vi "Configure Switcher Sweep Input.vi"(0 "VISA resource name":refnum<visa-resource-name>, 1 "Network Name (0)":string="0", 2 "Switch Number Of Steps (0)":i32, 5 "Channel (0: Channel A)":i32(ring) items=["Channel A", "Channel B"], 7 "Enable Input Switch (T: Enable)":bool=TRUE, 9 "Starting Logical Channel (0)":i32, 11 "error in (no error)":errorcluster, 12 "Switch Step Size (0)":i32) -> (4 "VISA resource name out":refnum<visa-resource-name>, 15 "error out":errorcluster)   [LabVIEW 2014, in "Stanford Research SR1.lvlib"]
doc: "Configures the attributes for the Switcher Sweep Input."
uses:
  Stanford Research SR1.lvlib
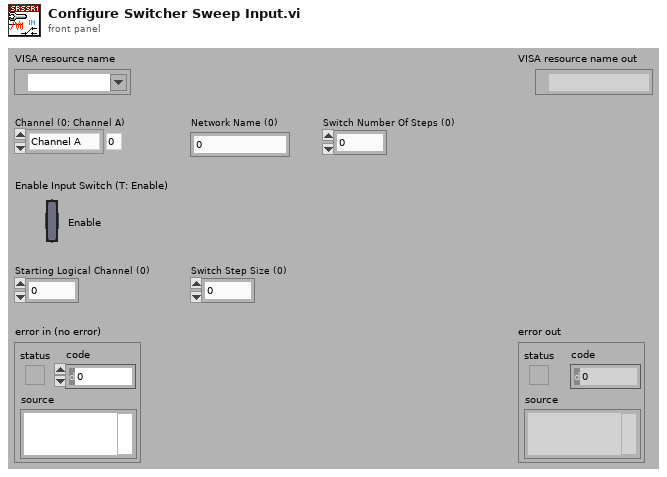
[diagram p1: front panel]
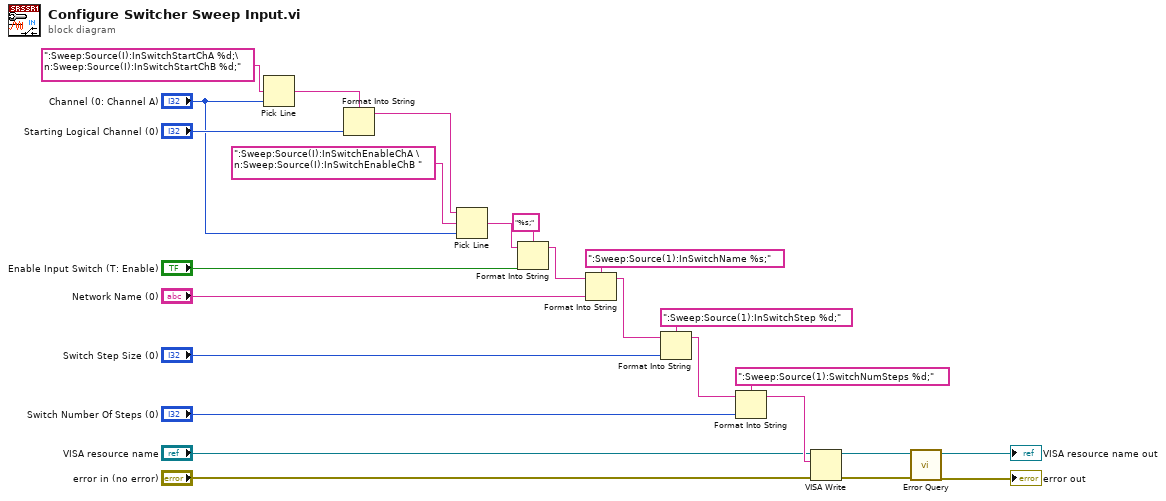
[diagram p0: block diagram]
diagram:
  n1 = Pick Line(multi-line string=":Sweep:Source(I):InSwitchStartChA %d;\n:Sweep:Source(I):InSwitchStartChB %d;", line index="Channel (0: Channel A)") -> (output string=w1:string)  [unwired: 1 in]
  n2 = Format Into String(format string=w1, "Starting Logical Channel (0)") -> (resulting string=w2:string)  [unwired: 2 in, 1 out]
  n3 = Pick Line(string ("")=w2, multi-line string=":Sweep:Source(I):InSwitchEnableChA \n:Sweep:Source(I):InSwitchEnableChB ", line index="Channel (0: Channel A)") -> (output string=w6:string)
  n4 = Format Into String(format string="%s;", initial string=w6, "Enable Input Switch (T: Enable)") -> (resulting string=w4:string)  [unwired: 1 in, 1 out]
  n5 = Format Into String(format string=":Sweep:Source(1):InSwitchName %s;", initial string=w4, "Network Name (0)") -> (resulting string=w23:string)  [unwired: 1 in, 1 out]
  n6 = Format Into String(format string=":Sweep:Source(1):InSwitchStep %d;", initial string=w23, "Switch Step Size (0)") -> (resulting string=w20:string)  [unwired: 1 in, 1 out]
  n7 = Format Into String(format string=":Sweep:Source(1):SwitchNumSteps %d;", initial string=w20, "Switch Number Of Steps (0)") -> (resulting string=w17:string)  [unwired: 1 in, 1 out]
  n8 = VISA Write(VISA resource name="VISA resource name", write buffer=w17, error in (no error)="error in (no error)") -> (VISA resource name out=w14:refnum<visa-resource-name>, error out=w13:errorcluster)  [unwired: 1 out]
  n9 = call "Error Query.vi"("error in (no error)"=w13, "VISA resource name"=w14) -> ("error out"=→"error out":errorcluster, "VISA resource name out"=→"VISA resource name out":refnum<visa-resource-name>)  [unwired: 6 in, 2 out]
